vi "Periodic Tasks.vi"(8 "error in":errorcluster) -> ()   [LabVIEW 2016]
doc: "This VI runs in parallel to other tasks. It can contain as many user-defined periodic loops as you need. These can carry out PID or other sorts of timed response."
uses:
  <vilib>/Rock Robotics/WPI/Utilities/WPI_GetSetVariantRefNum.vi
  <vilib>/Instr/_visa.llb/VISA Configure Serial Port (Instr).vi
  2_11_17/Systems/Global 1.vi
  <vilib>/Analysis/NI_AALBase.lvlib
  <vilib>/Analysis/3filter.llb/IIR Filter (DBL).vi
panel:
  in  "off set":dbl=55.0 format="%#_13g"
  out "read buffer":string="B:3,X:197.00,Y:124.00"
  in  "Search_Params":string[](array[string])=["B", "X", "Y", "W1", "H1", "W2", "H2"]
  out "Last Complete Message":string="B:2,X:197.00,Y:124.00,W1:9,H1:24,W2:9,H2:23"
  out "length":i32=43
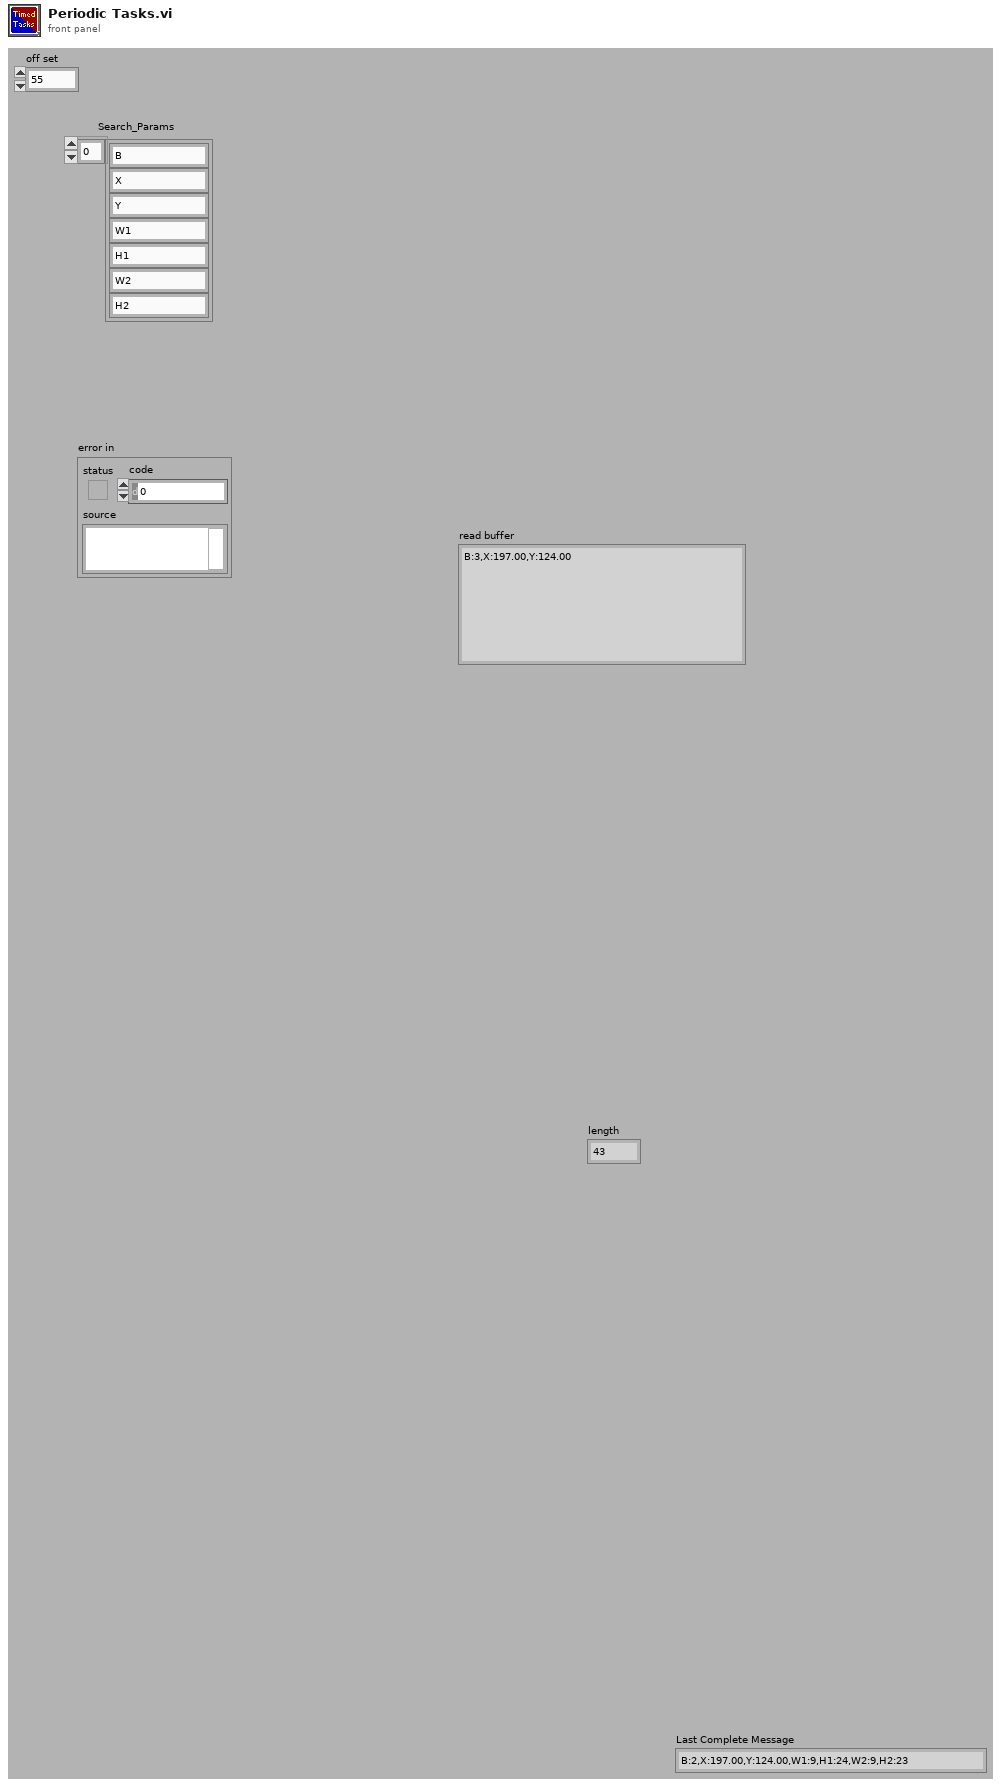
[diagram p1: front panel]
types:
  T1 = typedef "WPI_JoystickDevRef.ctl" = cluster{"Device":T2}
  T2 = typedef "WPI_JoystickDeviceEnum.ctl" = enum16{"USB 0", "USB 1", "USB 2", "USB 3", "USB 4", "USB 5"}
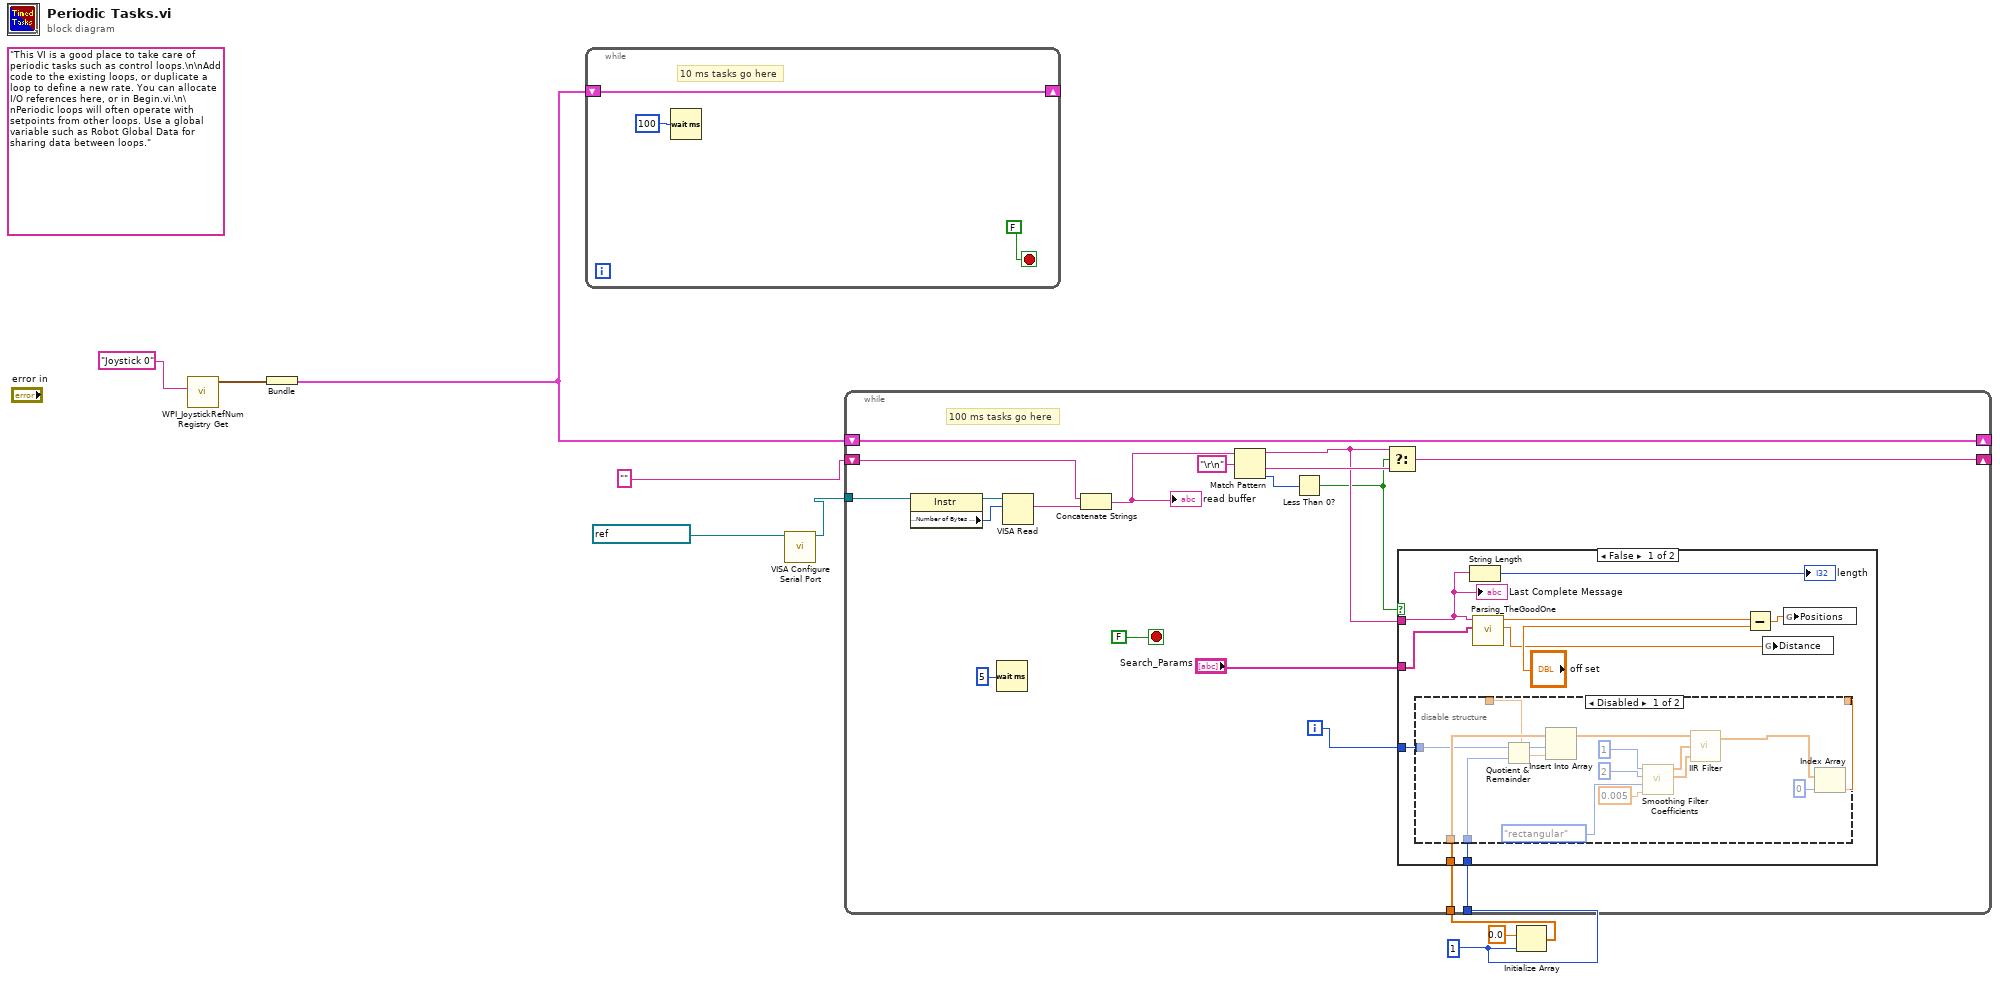
[diagram p0: block diagram]
diagram:
  w6 = 1
  (unwired) "This VI is a good place to take care of periodic tasks such as control loops.\n\nAdd code to the existing loops, or duplicate a loop to define a new rate. You can allocate I/O references here, or in Begin.vi.\n\nPeriodic loops will often operate with setpoints from other loops. Use a global variable such as Robot Global Data for sharing data between loops."
  n1 = call <vilib>:"WPI_JoystickRefNum Registry Get.vi"("refnum name"="Joystick 0") -> ("JoystickDevRef"=w8:T1)  [unwired: 1 in, 9 out]
  n2 = Bundle("JoystickDevRef"=w8) -> (w7:cluster{"JoystickDevRef":T1})  [unwired: 1 out]
  n3 = while {
    shift-right: [w10] -> _
    shift-left: w7 -> [w10]
    stop <- FALSE stop-if-true
    # "10 ms tasks go here"
    n4 = Wait (ms)(milliseconds to wait=u32 100) -> ()  [unwired: 1 out]
  }
  n5 = call-poly "VISA Configure Serial Port"("VISA resource name"=refnum<visa-resource-name> "ASRL2::INSTR") -> ("VISA resource name out"=w2:refnum<visa-resource-name>)  [unwired: 13 in, 1 out]
  n6 = Initialize Array(0.0 ("element"), w6) -> (w5:dbl[])
  n7 = while {
    shift-right: [w30] -> _
    shift-left: w7 -> [w30]
    tunnel: w2 -> [w25]
    shift-right: [w17] -> _
    shift-left: "" -> [w24]
    tunnel: w5 -> [w15]
    tunnel: w6 -> [w14]
    i -> [w13]
    stop <- FALSE stop-if-true
    # "100 ms tasks go here"
    n8 = property class="Instr"(reference=w25) -> (reference out=w29:refnum<visa-resource-name>, "Serial Settings:Number of Bytes at Serial Port"=w28:u32)  [unwired: 1 in, 1 out]
    n9 = Wait (ms)(milliseconds to wait=u32 5) -> ()  [unwired: 1 out]
    n10 = VISA Read(VISA resource name=w29, byte count=w28) -> (read buffer=w23:string)  [unwired: 1 in, 3 out]
    n11 = Concatenate Strings(w24, w23) -> (w22:string)
    "read buffer" <- w22
    n12 = Match Pattern(string=w22, regular expression="\r\n") -> (before substring=w18:string, after substring=w19:string, offset past match=w20:i32)  [unwired: 1 in, 1 out]
    n13 = Less Than 0?(x=w20) -> (x < 0?=w16:bool)
    n14 = Select(t=w18, s=w16, f=w19) -> (s? t:f=w17:string)
    n15 = case shown="False" w16 {
      tunnel: "Search_Params" -> [w40 _]
      tunnel: w18 -> [w39 _]
      tunnel: w15 -> [w35 _]
      tunnel: w14 -> [w34 _]
      tunnel: w13 -> [w33 _]
      frame False {
        n16 = disable-structure shown="Disabled" {
          disable-tunnel: w35 -> [w48 _]
          disable-tunnel: w34 -> [w47 _]
          disable-tunnel: w33 -> [w46 _]
          disable-tunnel: _ -> [w45 _]
          disable-tunnel: [w42 _] -> _
          frame Disabled {
            n17 = Quotient & Remainder(x=w46, y=w47) -> (x-y*floor(x/y)=w49:i32)  [unwired: 1 out]
            n18 = Insert Into Array(array=w48, index=w49, new element=w45) -> (w50:dbl[])
            n19 = call <vilib>:"Smoothing Filter Coefficients.vi"("time constant"=0.005, "shape"=enum16{"rectangular", "triangular"}."rectangular", "half-width"=2, "type"=1) -> ("forward coefficients"=w52:dbl[], "reverse coefficients"=w53:dbl[])  [unwired: 5 in, 1 out]
            n20 = call-poly <vilib>:"IIR Filter.vi"("Forward Coefficients"=w52, "Reverse Coefficients"=w53, "X"=w50) -> ("Filtered X"=w44:dbl[])  [unwired: 1 in, 1 out]
            n21 = Index Array(array=w44, index=0) -> (element=w42:dbl)
          }
          frame Enabled {
          }
        }
        n22 = String Length(string=w39) -> (length=→"length":i32)
        n23 = call "Parsing_TheGoodOne.vi"("Search_Params"=w40, "Input"=w39) -> ("Corrected distance"=w32:dbl, "Value-Reference"=w38:dbl)  [unwired: 6 in]
        n24 = Subtract(x=w38, y="off set") -> (x-y=w36:dbl)
        n25 = global write "Global 1.vi" "Distance"(w32) -> ()
        n26 = global write "Global 1.vi" "Positions"(w36) -> ()
        "Last Complete Message" <- w39
      }
      frame True {
      }
    }
  }
